vi "NI.AI_Freq.vi"(7 "input terminal configuration":i32(ring)=-1 caption="输入接线端配置" items=["默认"=-1, "RSE"=10083, "NRSE"=10078, "差分"=10106, "伪差分"=12529], 8 "error in":errorcluster caption="错误输入", 9 "SignalFreq":dbl=1000.0 min=1.0, 10 "AI Channel":T1(ring), 11 "DAQmx设备名":tag) -> (0 "error out":errorcluster caption="错误输出", 1 "MAX(V)":dbl, 2 "RMS(VDC)":dbl, 3 "VPP(V)":dbl, 4 "波形图":waveform(dbl)(graph), 5 "FREQ(Hz)":dbl, 6 "RMS(VAC)":dbl)   [LabVIEW 2012, in "Lib_UEL.ATE.lvlib" / "Lib_PCI6221.lvlib"]
uses:
  Lib_PCI6221.lvlib
  <vilib>/DAQmx/read.llb/DAQmx Read (Analog Wfm 1Chan NSamp).vi
  <vilib>/DAQmx/create/channels.llb/DAQmx Create Channel (AI-Voltage-Basic).vi
  <vilib>/DAQmx/configure/timing.llb/DAQmx Timing (Sample Clock).vi
  <vilib>/DAQmx/miscellaneous.llb/DAQmx Fill In Error Info.vi
panel:
  in  "测试日志信息 2":refnum<queue>
  # "V01 - Initial Version.  ~ LiGuang 2011-05-12\n        - Default, 波形图会显示四个周期 \nV02 - 2013/1/11, 增加日志功能: 将操作信息压入到输入的队列中.\nV03 - 2013/3/23, LiGuang, 增加Vrms(AC)计算,区分直流和交流有效值."
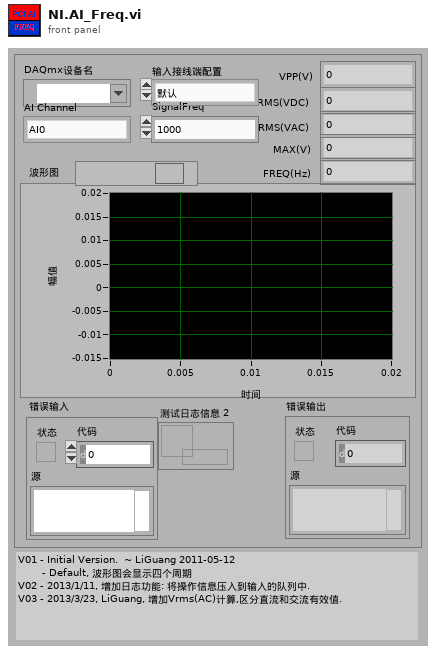
[diagram p1: front panel]
types:
  T1 = enum16{"AI0", "AI1", "AI2", "AI3", "AI4", "AI5", "AI6", "AI7", "AI8", "AI9", "AI10", "AI11", "AI12", "AI13", "AI14", "AI15"}
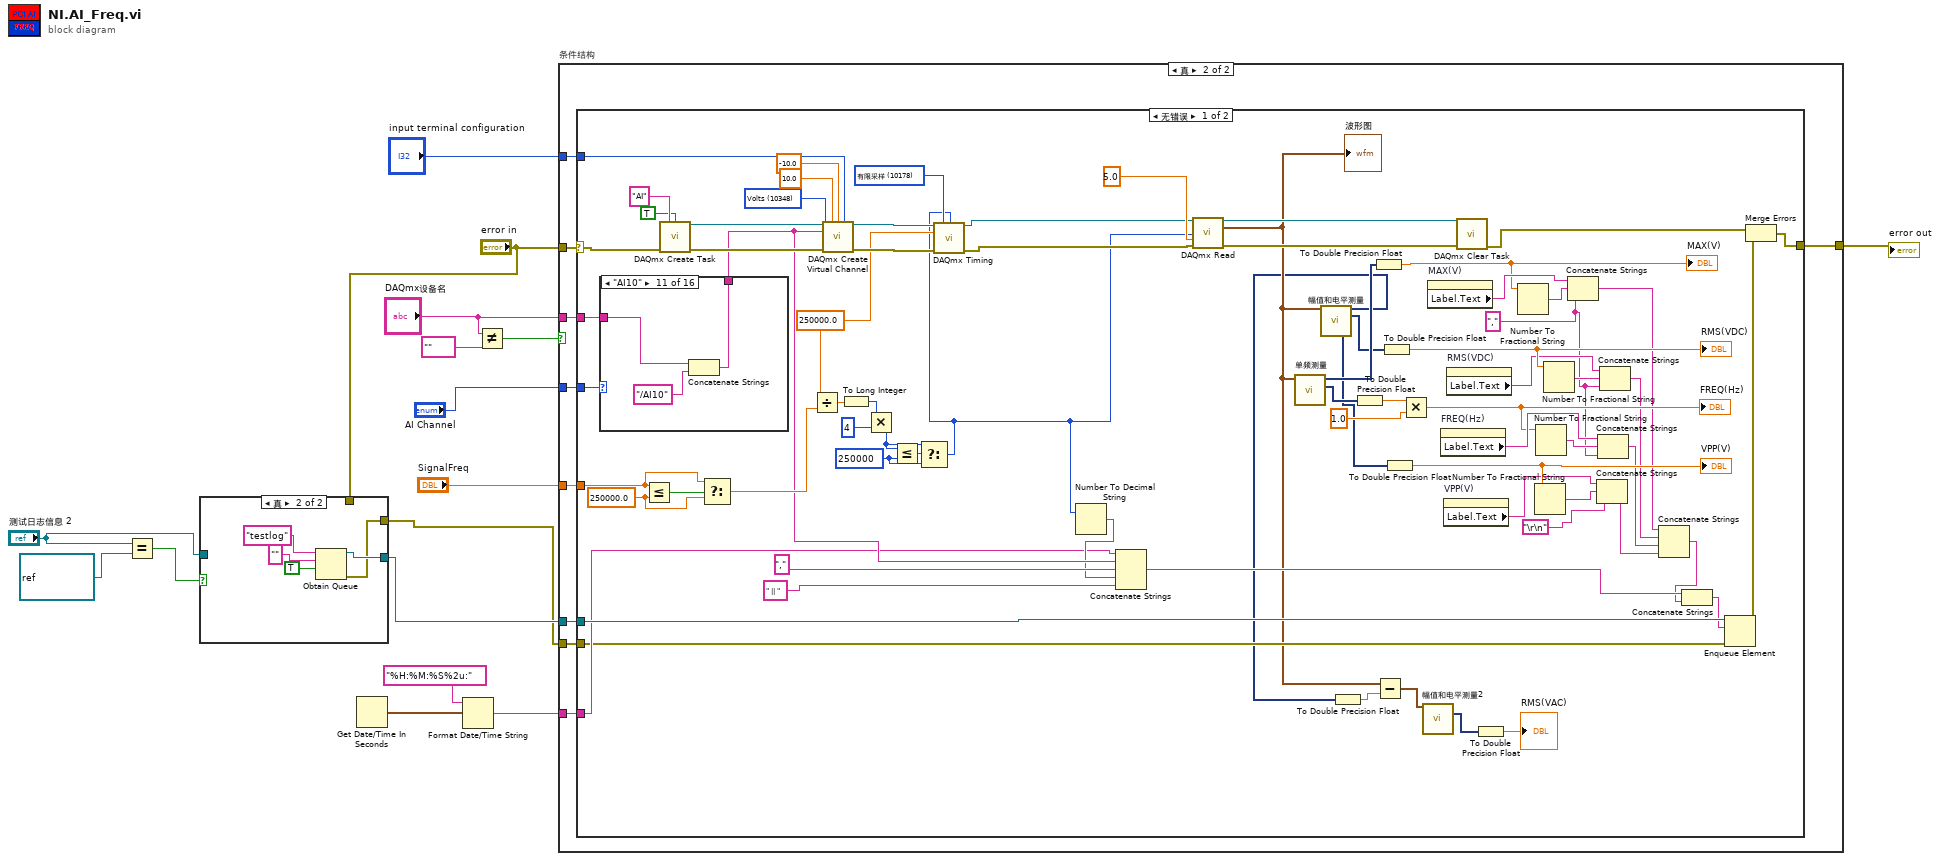
[diagram p0: block diagram]
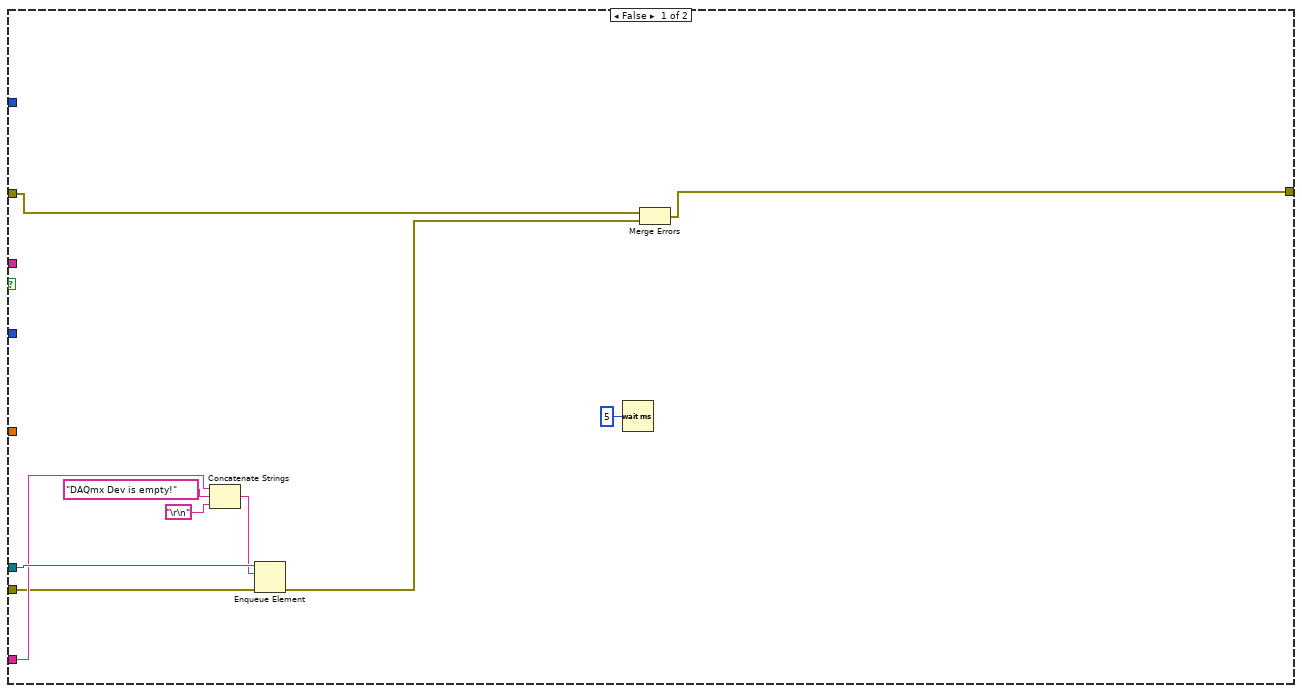
[diagram p3: hidden frame]
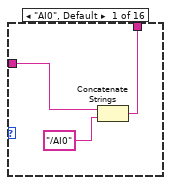
[diagram p4: hidden frame]
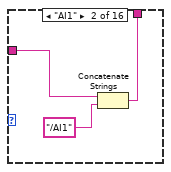
[diagram p5: hidden frame]
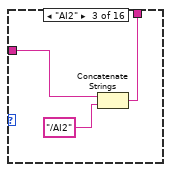
[diagram p6: hidden frame]
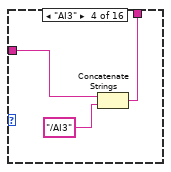
[diagram p7: hidden frame]
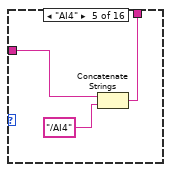
[diagram p8: hidden frame]
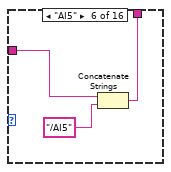
[diagram p9: hidden frame]
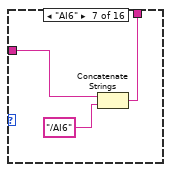
[diagram p10: hidden frame]
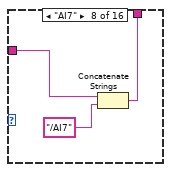
[diagram p11: hidden frame]
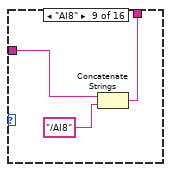
[diagram p12: hidden frame]
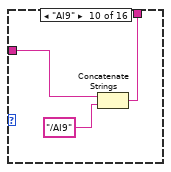
[diagram p13: hidden frame]
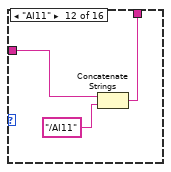
[diagram p14: hidden frame]
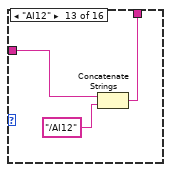
[diagram p15: hidden frame]
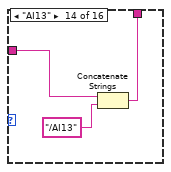
[diagram p16: hidden frame]
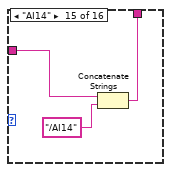
[diagram p17: hidden frame]
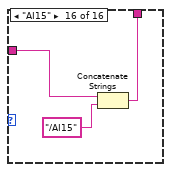
[diagram p18: hidden frame]
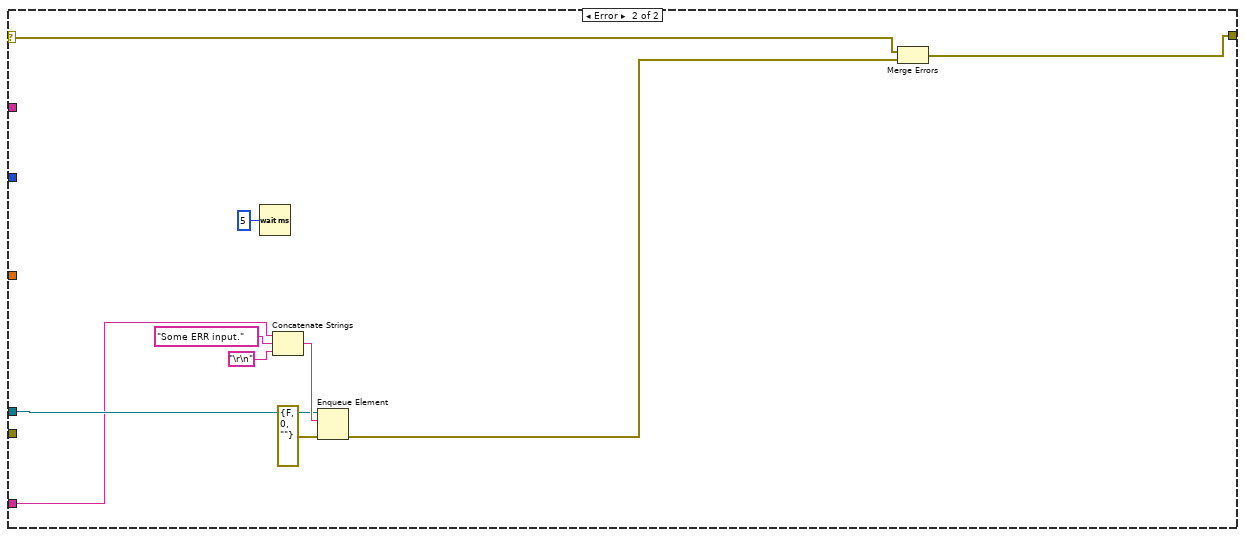
[diagram p19: hidden frame]
diagram:
  n1 = Equal?(x="测试日志信息 2", y=refnum<queue> refnum ("测试日志信息")) -> (x = y?=w5:bool)
  n2 = case shown="真" w5 {
    tunnel: "测试日志信息 2" -> [w18 _]
    tunnel: [w18 w23] -> w3
    tunnel: [w17 w19] -> w2
    tunnel: "error in" -> [w17 _]
    frame False {
    }
    frame True {
      n3 = Obtain Queue(name (unnamed)="testlog" ("名称（未命名）"), element data type="" ("名称（未命名）"), create if not found? (T)=TRUE ("如未找到是否创建？(T)")) -> (queue out=w23:refnum<queue>, error out=w19:errorcluster)  [unwired: 2 in, 1 out]
    }
  }
  n4 = Get Date/Time In Seconds() -> (seconds since 1Jan1904=w8:timestamp)
  n5 = Format Date/Time String(time format string (%c)="%H:%M:%S%2u:" ("时间格式化字符串(%c)"), seconds (now)=w8) -> (date/time string=w7:string)  [unwired: 1 in]
  n6 = Not Equal?(x="DAQmx设备名", y=tag "") -> (x != y?=w11:bool)
  n7 = case "条件结构" shown="真" w11 {
    tunnel: "error in" -> [w28 w42]
    tunnel: [w26 w41] -> w16
    tunnel: "SignalFreq" -> [_ w40]
    tunnel: "AI Channel" -> [_ w39]
    tunnel: "DAQmx设备名" -> [_ w38]
    tunnel: "input terminal configuration" -> [_ w37]
    tunnel: w3 -> [w33 w36]
    tunnel: w7 -> [w29 w35]
    tunnel: w2 -> [w24 w34]
    frame False {
      n8 = Concatenate Strings(w29, "DAQmx Dev is empty!" ("元素"), "\r\n") -> (w30:string)
      n9 = Enqueue Element(queue=w33, element=w30, error in (no error)=w24) -> (error out=w27:errorcluster)  [unwired: 1 in, 2 out]
      n10 = Wait (ms)(milliseconds to wait=u32 5 ("等待时间（毫秒）")) -> ()  [unwired: 1 out]
      n11 = Merge Errors(w28, w27) -> (w26:errorcluster)
    }
    frame True {
      n12 = case shown="无错误" w42 {
        selector: w42 -> [w116 w166]
        tunnel: [w92 w165] -> w41
        tunnel: w40 -> [w105 _]
        tunnel: w39 -> [w107 _]
        tunnel: w38 -> [w101 _]
        tunnel: w37 -> [w98 _]
        tunnel: w36 -> [w95 w171]
        tunnel: w35 -> [w67 w170]
        tunnel: w34 -> [w66 _]
        frame No Error {
          w56 = 250000 ("y")
          w104 = 250000.0 ("y")
          w99 = 250000.0 ("rate")
          w61 = 10178 items=["有限采样"=10178, "连续采样"=10123, "硬件定时单点"=12522] ("sample mode")
          w79 = "," ("时间格式化字符串(%c)")
          w110 = 10348 items=["Volts"=10348, "来自自定义换算"=10065] ("units")
          n13 = case shown="\"AI10\"" w107 {
            tunnel: [w117 w120 w123 w126 w129 w132 w135 w138 w141 w144 w147 w150 w153 w156 w159 w162] -> w91
            tunnel: w101 -> [w118 w121 w124 w127 w130 w133 w136 w139 w142 w145 w148 w151 w154 w157 w160 w163]
            frame "AI0", Default {
              n14 = Concatenate Strings(w118, "/AI0") -> (w117:string)
            }
            frame "AI1" {
              n15 = Concatenate Strings(w121, "/AI1") -> (w120:string)
            }
            frame "AI2" {
              n16 = Concatenate Strings(w124, "/AI2") -> (w123:string)
            }
            frame "AI3" {
              n17 = Concatenate Strings(w127, "/AI3") -> (w126:string)
            }
            frame "AI4" {
              n18 = Concatenate Strings(w130, "/AI4") -> (w129:string)
            }
            frame "AI5" {
              n19 = Concatenate Strings(w133, "/AI5") -> (w132:string)
            }
            frame "AI6" {
              n20 = Concatenate Strings(w136, "/AI6") -> (w135:string)
            }
            frame "AI7" {
              n21 = Concatenate Strings(w139, "/AI7") -> (w138:string)
            }
            frame "AI8" {
              n22 = Concatenate Strings(w142, "/AI8") -> (w141:string)
            }
            frame "AI9" {
              n23 = Concatenate Strings(w145, "/AI9") -> (w144:string)
            }
            frame "AI10" {
              n24 = Concatenate Strings(w148, "/AI10") -> (w147:string)
            }
            frame "AI11" {
              n25 = Concatenate Strings(w151, "/AI11") -> (w150:string)
            }
            frame "AI12" {
              n26 = Concatenate Strings(w154, "/AI12") -> (w153:string)
            }
            frame "AI13" {
              n27 = Concatenate Strings(w157, "/AI13") -> (w156:string)
            }
            frame "AI14" {
              n28 = Concatenate Strings(w160, "/AI14") -> (w159:string)
            }
            frame "AI15" {
              n29 = Concatenate Strings(w163, "/AI15") -> (w162:string)
            }
          }
          n30 = Less Or Equal?(x=w105, y=w104) -> (x <= y?=w106:bool)
          n31 = call <vilib>:"DAQmx Create Task.vi"("new task name"="AI", "auto cleanup"=TRUE, "error in"=w116) -> ("task out"=w114:refnum<k21>, "error out"=w113:errorcluster)  [unwired: 11 in]
          n32 = Select(t=w105, s=w106, f=w104) -> (s? t:f=w103:dbl)
          n33 = Divide(x=w99, y=w103) -> (x/y=w64:dbl)
          n34 = call-poly <vilib>:"DAQmx Create Virtual Channel.vi"("task in"=w114, "maximum value"=10.0, "minimum value"=-10.0, "input terminal configuration"=w98, "physical channels"=w91, "units"=w110, "error in"=w113) -> ("task out"=w109:refnum<k21>, "error out"=w108:errorcluster)  [unwired: 7 in]
          n35 = To Long Integer(number=w64) -> (32bit integer=w60:i32)
          n36 = Multiply(x=w60, y=4) -> (x*y=w57:i32)
          n37 = Less Or Equal?(x=w57, y=w56) -> (x <= y?=w58:bool)
          n38 = Select(t=w57, s=w58, f=w56) -> (s? t:f=w55:i32)
          n39 = call-poly <vilib>:"DAQmx Timing.vi"("task/channels in"=w109, "sample mode"=w61, "samples per channel"=w55, "rate"=w99, "error in"=w108) -> ("task out"=w63:refnum<k21>, "error out"=w62:errorcluster)  [unwired: 9 in]
          n40 = Number To Decimal String(number=w55) -> (decimal integer string=w89:string)  [unwired: 1 in]
          n41 = Concatenate Strings(w67, w91, "," ("时间格式化字符串(%c)"), w89, " || " ("时间格式化字符串(%c)")) -> (w70:string)
          n42 = call-poly <vilib>:"DAQmx Read.vi"("task/channels in"=w63, "number of samples per channel"=w55, "timeout"=5.0, "error in"=w62) -> ("task out"=w112:refnum<k21>, "data"=w54:waveform(dbl), "error out"=w111:errorcluster)  [unwired: 9 in]
          "波形图" <- w54
          n43 = call "单频测量"("Signals"=w54) -> ("Frequency"=w51:dynamicdata, "Amplitude"=w52:dynamicdata)  [unwired: 8 in, 1 out]
          n44 = call "幅值和电平测量"("Signals"=w54) -> ("Mean (DC)"=w46:dynamicdata, "RMS"=w45:dynamicdata, "Peak to Peak"=w44:dynamicdata)  [unwired: 11 in, 1 out]
          n45 = To Double Precision Float(number=w46) -> (double precision float=w48:dbl)
          n46 = To Double Precision Float(number=w51) -> (double precision float=w50:dbl)
          n47 = To Double Precision Float(number=w52) -> (double precision float=w47:dbl)
          "MAX(V)" <- w47
          n48 = Subtract(x=w54, y=w48) -> (x-y=w53:waveform(dbl))
          n49 = To Double Precision Float(number=w45) -> (double precision float=w85:dbl)
          "RMS(VDC)" <- w85
          n50 = To Double Precision Float(number=w44) -> (double precision float=w78:dbl)
          "VPP(V)" <- w78
          n51 = Multiply(x=w50, y=1.0 ("rate")) -> (x*y=w80:dbl)
          "FREQ(Hz)" <- w80
          n52 = call "幅值和电平测量2"("Signals"=w53) -> ("RMS"=w43:dynamicdata)  [unwired: 13 in, 1 out]
          n53 = property on="MAX(V)" class="DigNum (严格)"() -> ("Label.Text"=w87:string)  [unwired: 2 in, 2 out]
          n54 = property on="FREQ(Hz)" class="DigNum (严格)"() -> ("Label.Text"=w82:string)  [unwired: 2 in, 2 out]
          n55 = property on="VPP(V)" class="DigNum (严格)"() -> ("Label.Text"=w77:string)  [unwired: 2 in, 2 out]
          n56 = property on="RMS(VDC)" class="DigNum (严格)"() -> ("Label.Text"=w84:string)  [unwired: 2 in, 2 out]
          n57 = call <vilib>:"DAQmx Clear Task.vi"("task in"=w112, "error in"=w111) -> ("error out"=w94:errorcluster)  [unwired: 13 in]
          n58 = To Double Precision Float(number=w43) -> (double precision float=→"RMS(VAC)":dbl)
          n59 = Number To Fractional String(number=w47) -> (F-format string=w86:string)  [unwired: 3 in]
          n60 = Number To Fractional String(number=w78) -> (F-format string=w76:string)  [unwired: 3 in]
          n61 = Number To Fractional String(number=w80) -> (F-format string=w81:string)  [unwired: 3 in]
          n62 = Number To Fractional String(number=w85) -> (F-format string=w83:string)  [unwired: 3 in]
          n63 = Concatenate Strings(w87, w86, w79) -> (w74:string)
          n64 = Concatenate Strings(w77, w76, "\r\n") -> (w71:string)
          n65 = Concatenate Strings(w82, w81, w79) -> (w72:string)
          n66 = Concatenate Strings(w84, w83, w79) -> (w73:string)
          n67 = Concatenate Strings(w74, w73, w72, w71) -> (w69:string)
          n68 = Concatenate Strings(w70, w69) -> (w68:string)
          n69 = Enqueue Element(queue=w95, element=w68, error in (no error)=w66) -> (error out=w93:errorcluster)  [unwired: 1 in, 2 out]
          n70 = Merge Errors(w94, w93) -> (w92:errorcluster)
        }
        frame Error {
          n71 = Wait (ms)(milliseconds to wait=u32 5 ("等待时间（毫秒）")) -> ()  [unwired: 1 out]
          n72 = Concatenate Strings(w170, "Some ERR input." ("元素"), "\r\n") -> (w172:string)
          n73 = Enqueue Element(queue=w171, element=w172, error in (no error)=errorcluster {"status"=FALSE, "code"=0, "source"=""} ("错误输入（无错误）")) -> (error out=w167:errorcluster)  [unwired: 1 in, 2 out]
          n74 = Merge Errors(w166, w167) -> (w165:errorcluster)
        }
      }
    }
  }
  "error out" <- w16
